vi "XIPIN_SMPTE_SD_HD_3G-SDI_3_0.vi"   [LabVIEW 2017]
doc: "SMPTE Serial Digital Interface carries uncompressed digital video and ancillary data\n------------------------------------\n<b>Need License</b> : No"
uses:
  <vilib>/rvi/XilinxIP/XIPIN_XNode/niFpgaXIPIN.xnode
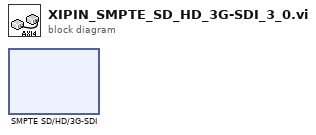
[diagram p0: block diagram]
diagram:
  n1 = xnode ("SMPTE SD/HD/3G-SDI")() -> ()
